vi "Send timing status.vi"(8 "error in (no error)":errorcluster, 10 "out of time?":bool, 11 "DAQOrcaFlash in":refnum<class "DAQOrcaFlash.lvclass">) -> (0 "error out":errorcluster, 3 "DAQOrcaFlash out":refnum<class "DAQOrcaFlash.lvclass">)   [LabVIEW 2012, in "DAQOrcaFlash.lvclass"]
uses:
  DAQOrcaFlash.lvclass
  <vilib>/Distrio/Murmex/Murmex/Murmex.lvclass
  <vilib>/Distrio/Murmex/GenericMessage/GenericMessage.lvclass
  <vilib>/Distrio/Murmex/Message/Message.lvclass
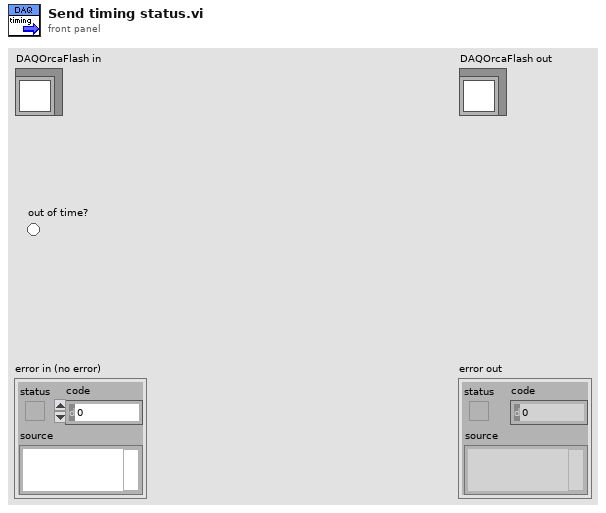
[diagram p1: front panel]
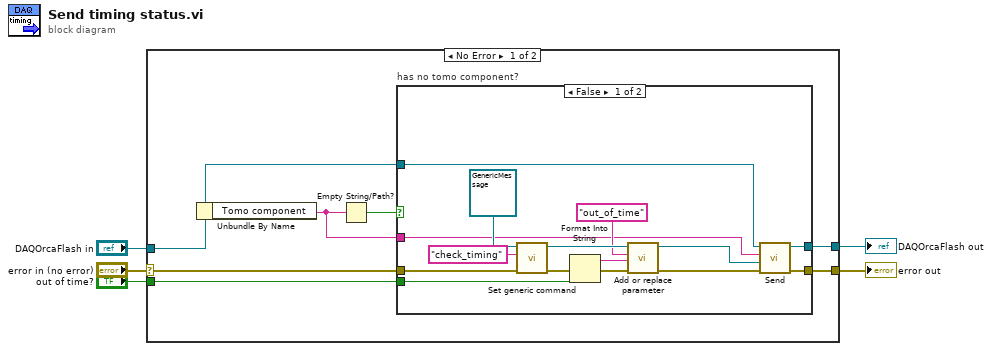
[diagram p0: block diagram]
diagram:
  n1 = case shown="No Error" "error in (no error)" {
    selector: "error in (no error)" -> [w6 w31]
    tunnel: [w7 w31] -> w4
    tunnel: [w8 w30] -> w2
    tunnel: "DAQOrcaFlash in" -> [w9 w30]
    tunnel: "out of time?" -> [w11 _]
    frame No Error {
      n2 = Unbundle By Name(w9) -> ("Tomo component"=w10:string)
      n3 = Empty String/Path?(string/path=w10) -> (empty?=w12:bool)
      n4 = case "has no tomo component?" shown="False" w12 {
        tunnel: w6 -> [w27 w29]
        tunnel: w11 -> [w18 _]
        tunnel: w10 -> [w16 _]
        tunnel: w9 -> [w15 w28]
        tunnel: [w14 w28] -> w8
        tunnel: [w13 w29] -> w7
        frame False {
          n5 = call <vilib>:"Set generic command.vi"("error in (no error)"=w27, "generic command"="check_timing", "GenericMessage in"=refnum<class "GenericMessage.lvclass"> refnum ("Distrio Murmex 1.5:GenericMessage")) -> ("error out"=w20:errorcluster, "GenericMessage out"=w22:refnum<class "GenericMessage.lvclass">)  [unwired: 7 in]
          n6 = Format Into String(error in=w20, w18) -> (resulting string=w17:string, error out=w19:errorcluster)  [unwired: 2 in]
          n7 = call <vilib>:"Add or replace parameter.vi"("error in (no error)"=w19, "value"=w17, "name"="out_of_time", "Message in"=w22) -> ("error out"=w24:errorcluster, "Message out"=w23:refnum<class "GenericMessage.lvclass">)  [unwired: 6 in]
          n8 = call <vilib>:"Send.vi"("error in (no error)"=w24, "Message"=w23, "recipient"=w16, "Murmex in"=w15) -> ("error out"=w13:errorcluster, "Murmex out"=w14:refnum<class "DAQOrcaFlash.lvclass">)  [unwired: 6 in]
        }
        frame True {
        }
      }
    }
    frame Error {
    }
  }
  "error out" <- w4
  "DAQOrcaFlash out" <- w2
